vi "Test Temperhum Inheritance.vi"() -> ()   [LabVIEW 2019, in "Instrument.Temperhum.lvclass"]
uses:
  Instrument.Temperhum.lvclass
  Temperhum.Thorlabs/Temperhum.Thorlabs.lvclass
  C:/Users/ansom/Documents/GitHub/Temperhum-Instrument/lvsrc/SMOs/Instrument.Temperhum/Instrument.Temperhum.lvclass
  Temperhum.PCSensor/Temperhum.PCSensor.lvclass
panel:
  in  "stop":bool
  out "Processed Data":variant
  out "x-y":dbl
  in  "Enum":enum16{"parent", "thorlabs", "pc sensor"}(ring)
  out "error out":errorcluster
  in  "error in (no error)":errorcluster
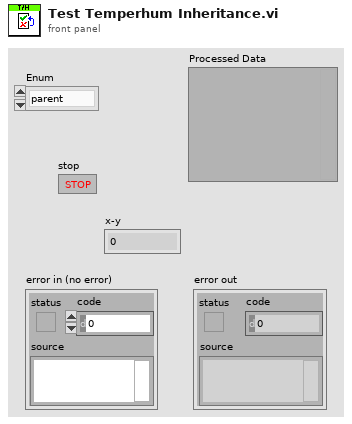
[diagram p1: front panel]
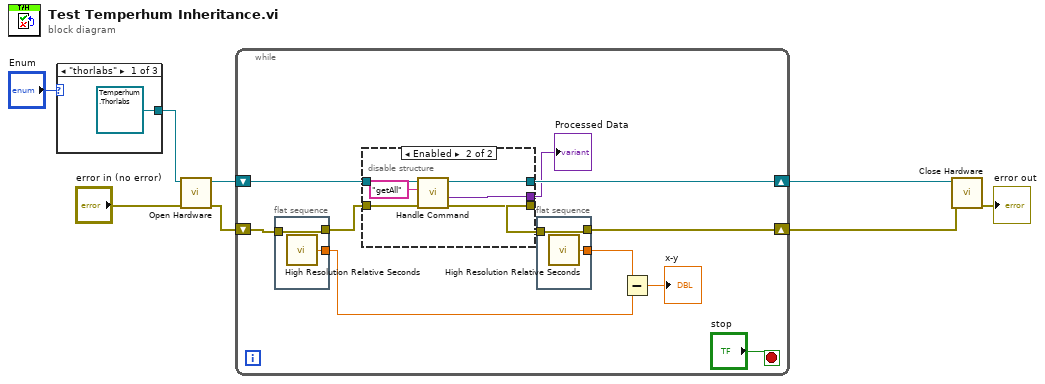
[diagram p0: block diagram]
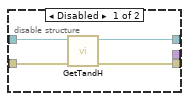
[diagram p2: hidden frame]
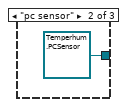
[diagram p3: hidden frame]
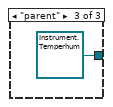
[diagram p4: hidden frame]
diagram:
  n1 = case shown="\"thorlabs\"" "Enum" {
    tunnel: [refnum<class "Temperhum.Thorlabs.lvclass"> refnum ("Temperhum.Thorlabs.lvclass") refnum<class "Temperhum.PCSensor.lvclass"> refnum ("Temperhum.PCSensor.lvclass") refnum<class "Instrument.Temperhum.lvclass"> refnum ("Instrument.Temperhum.lvclass")] -> w3
    frame "thorlabs" {
    }
    frame "pc sensor" {
    }
    frame "parent" {
    }
  }
  n2 = call-dynamic "Open Hardware.vi"("error in (no error)"="error in (no error)", "Instrument.FrameworkTemplate"=w3) -> ("error out"=w1:errorcluster, "Instrument.FrameworkTemplate out"=w8:refnum<class "Instrument.Temperhum.lvclass">)  [unwired: 8 in]
  n3 = while {
    shift-right: [w21] -> w7
    shift-left: w8 -> [w22]
    shift-right: [w20] -> w2
    shift-left: w1 -> [w13]
    stop <- "stop" stop-if-true
    n4 = flat-sequence {
      tunnel: w13 -> [w36]
      tunnel: [w36] -> w17
      tunnel: [w35] -> w15
      frame #0 {
        n5 = call <vilib>:"High Resolution Relative Seconds.vi"() -> ("relative seconds"=w35:dbl)
      }
    }
    n6 = disable-structure shown="Enabled" {
      disable-tunnel: w22 -> [w26 w32]
      disable-tunnel: [w25 w30] -> w21
      disable-tunnel: w17 -> [w24 w31]
      disable-tunnel: [w23 w29] -> w16
      disable-tunnel: [_ w27] -> w14
      frame Disabled {
        n7 = call-dynamic "GetTandH.vi"("error in (no error)"=w24, "Instrument.Temperhum in"=w26) -> ("error out"=w23:errorcluster, "Instrument.Temperhum out"=w25:refnum<class "Instrument.Temperhum.lvclass">)  [unwired: 6 in, 2 out]
      }
      frame Enabled {
        n8 = call-dynamic "Handle Command.vi"("error in (no error)"=w31, "Command"="getAll", "Instrument.FrameworkTemplate"=w32) -> ("error out"=w29:errorcluster, "Processed Data"=w27:variant, "Instrument.FrameworkTemplate out"=w30:refnum<class "Instrument.Temperhum.lvclass">)  [unwired: 5 in, 1 out]
      }
    }
    "Processed Data" <- w14
    n9 = flat-sequence {
      tunnel: w16 -> [w34]
      tunnel: [w34] -> w20
      tunnel: [w33] -> w19
      frame #0 {
        n10 = call <vilib>:"High Resolution Relative Seconds.vi"() -> ("relative seconds"=w33:dbl)
      }
    }
    n11 = Subtract(x=w19, y=w15) -> (x-y=→"x-y":dbl)
  }
  n12 = call-dynamic "Close Hardware.vi"("error in (no error)"=w2, "Instrument.FrameworkTemplate"=w7) -> ("error out"=→"error out":errorcluster)  [unwired: 8 in, 1 out]
